vi "motor_control.vi"(6 "Drive Motor Setpoint":fxp<+/-,16,32>, 7 "Steer Motor Setpoint":fxp<+/-,16,32>) -> (0 "Wheel Position 2":i32, 1 "Desired Drive Motor Speed":fxp<+/-,16,32>, 2 "Wheel Position":i32, 3 "Desired Steer Motor Speed":fxp<+/-,16,32>)   [LabVIEW 2009]
uses:
  <vilib>/Platform/TimedLoop/XDataNode/XDataNode.xnode
  <vilib>/Platform/TimedLoop/XDataNode/loadlvalarms.vi
  <vilib>/Platform/TimedLoop/XDataNode/timing_clust.ctl
  <vilib>/Platform/TimedLoop/XDataNode/nitl_modes.ctl
  <vilib>/Platform/TimedLoop/XDataNode/wakeup.ctl
  <vilib>/eio/EIONode/EIONode.xnode
  <vilib>/rvi/eio/nirviEIOImplementation/nirviEIOImplementation.xnode
  <vilib>/rvi/eio/common/nirviEmuTemplateMethod_noerrors.vi
  <vilib>/rvi/eio/common/nirviEmuClasses.ctl
  <vilib>/addons/control/pid/fpga.llb/XNode/niFpgaPID.xnode
  <vilib>/Platform/TimedLoop/XDataNode/XDNodeRunTimeDep.lvlib
panel:
  in  "M1 Reset Position 2":bool
  in  "M1 Reset Position Value 2":i32
  out "M1 Encoder Position 2":i32
  out "M1 ticks/count 2":u32
  out "M1 Index (Z) Position 2":i32
  out "M1 counts (no reset) 2":i32
  in  "M1 Reset Position":bool
  in  "M1 Reset Position Value":i32
  out "M1 Encoder Position":i32
  out "M1 ticks/count":u32
  out "M1 Index (Z) Position":i32
  out "M1 counts (no reset)":i32
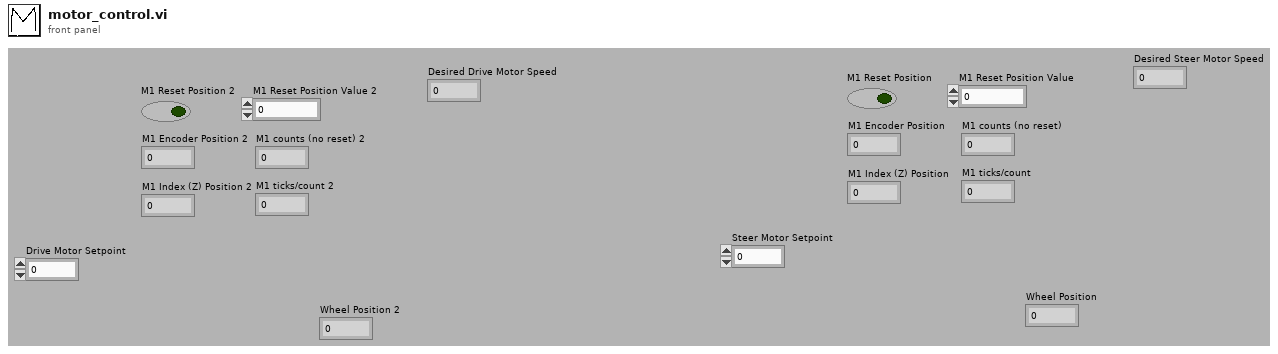
[diagram p1: front panel]
types:
  T1 = typedef "XDNodeRunTimeDep.lvlib/timing_clust.ctl" = cluster{"Expected End [f-1]":u64, "Actual End [f-1]":u64, "Finished Late? [f-1]":bool, "Expected End [i-1]":u64, "Actual End [i-1]":u64, "Finished Late? [i-1]":bool, "Expected Start [i]":u64, "Actual Start [i]":u64, "Expected Start [f]":u64, "Actual Start [f]":u64, "Source Name":string, "Structure Name":string, "Period":i64, "Deadline":i64, "Offset":i64, "Start":i64, "Priority":i32, "Timeout":i32, "Mode":T2, "Wakeup Reason":T3, "Error":errorcluster, "Source Type":string, "Secondary Source Type":string, "Global End Time":u64, "Global Start Time":u64, "Frame Duration":u64, "Iteration Duration":u64, "Assigned CPU":i32, "I/O Scan Engine Mode":u32}
  T2 = typedef "XDNodeRunTimeDep.lvlib/nitl_modes.ctl" = enum32{"No Change", "Process missed periods, maintain original phase", "Discard missed periods, maintain original phase", "Process missed periods, ignore original phase", "Discard missed periods, ignore original phase"}
  T3 = typedef "XDNodeRunTimeDep.lvlib/wakeup.ctl" = enum32{"Normal", "Aborted", "Asynchronous wakeup", "Timing source error", "Timed loop error", "Timeout"}
  T4 = cluster{"proportional gain (Kc)":i16, "integral gain (Kc*Ts/Ti)":i16, "derivative gain (Kc*Td/Ts)":i16}
  T5 = typedef "nirviEmuClasses.ctl" = enum16{"IO Read", "IO Write", "Method", "Property Read", "Property Write"}
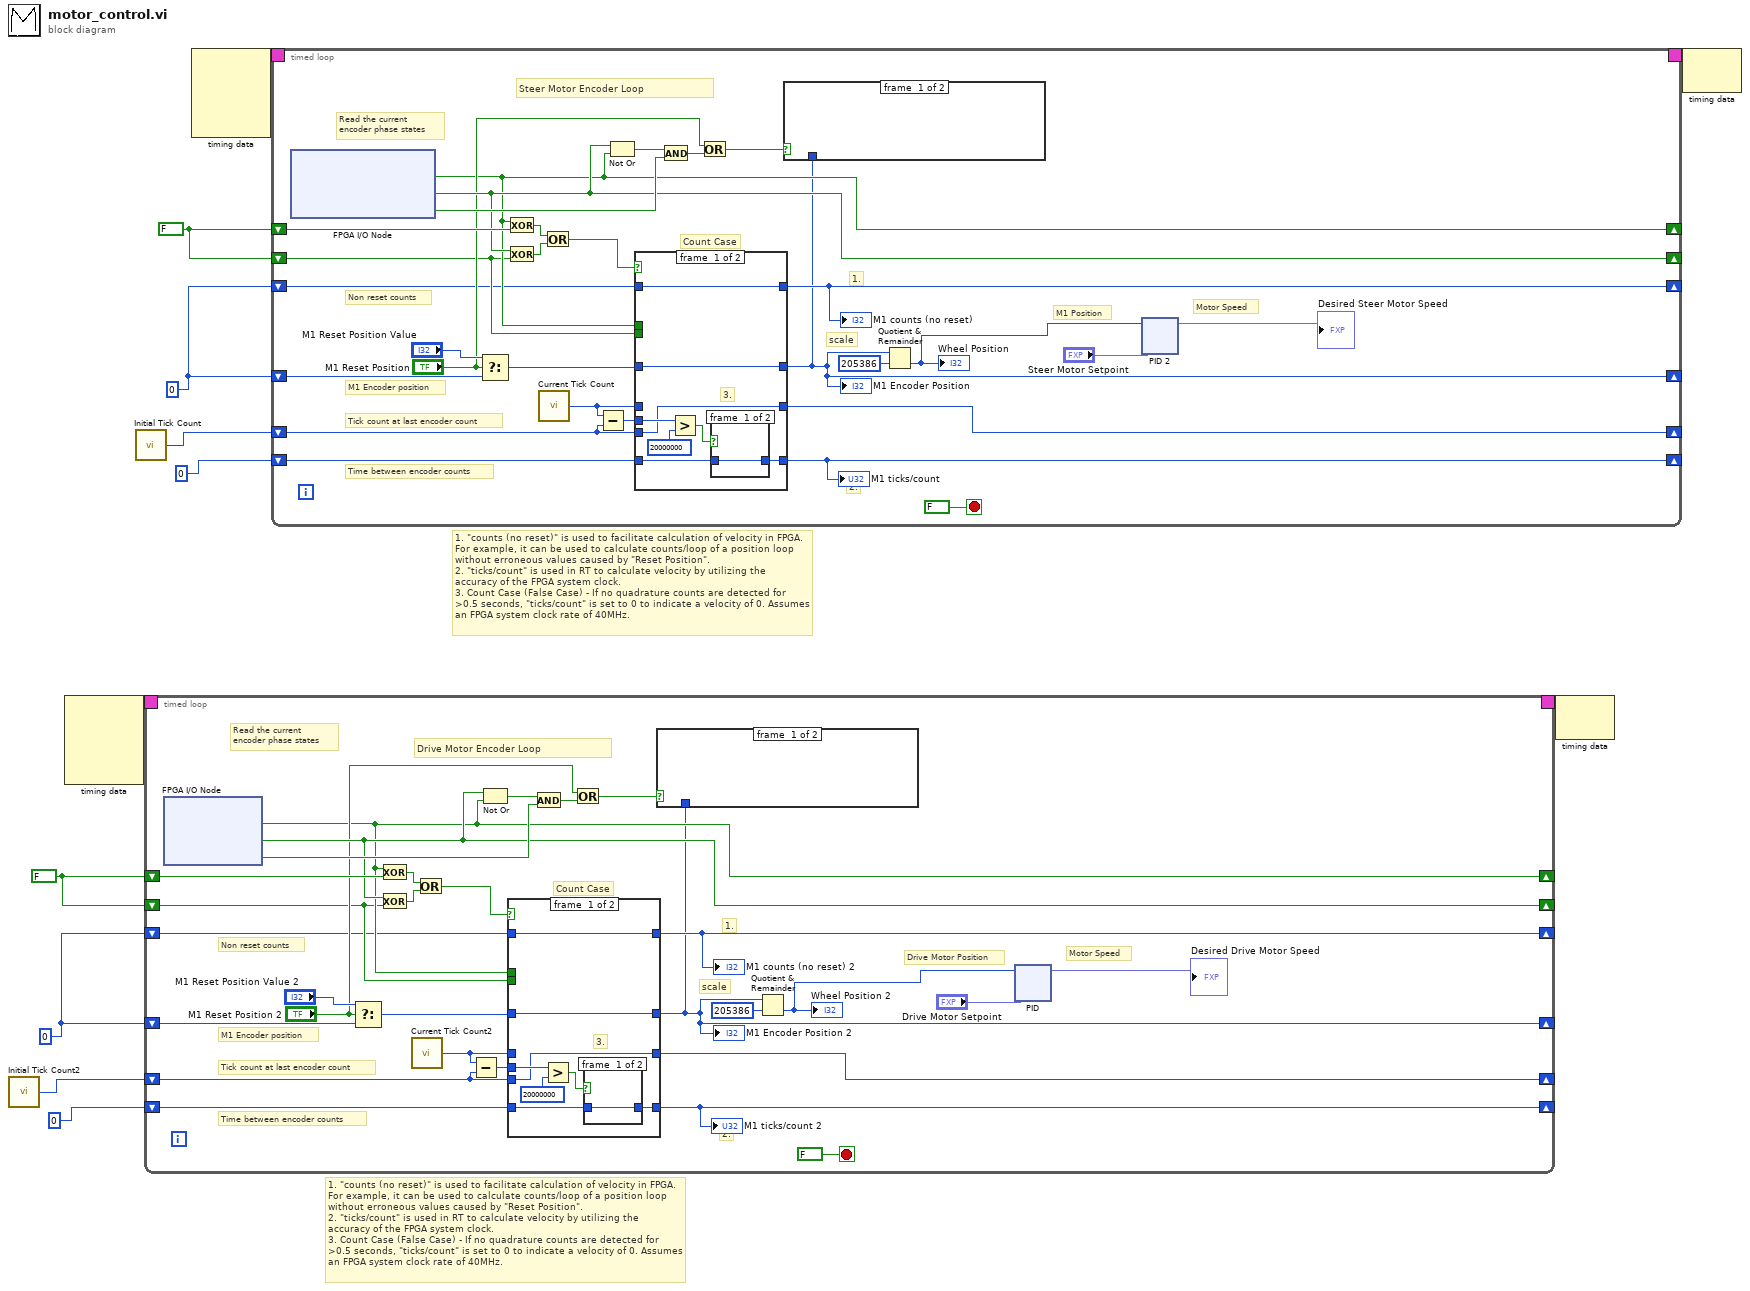
[diagram p0: block diagram]
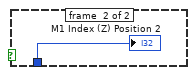
[diagram p2: hidden frame]
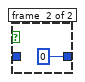
[diagram p3: hidden frame]
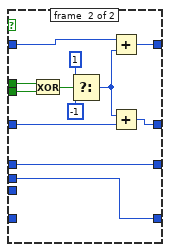
[diagram p4: hidden frame]
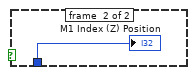
[diagram p5: hidden frame]
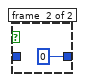
[diagram p6: hidden frame]
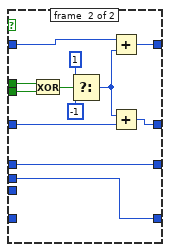
[diagram p7: hidden frame]
diagram:
  w1 = 0 ("Reset Position Value")
  w4 = FALSE ("Encoder Phase A")
  w7 = 0 ("Reset Position Value")
  w10 = FALSE ("Encoder Phase A")
  # "1. \"counts (no reset)\" is used to facilitate calculation of velocity in FPGA.\nFor example, it can be used to calculate counts/loop of a position loop\nwithout erroneous values caused by \"Reset Position\". \n2. \"ticks/count\" is used in RT to calculate velocity by utilizing the\naccuracy of the FPGA system clock.\n3. Count Case (False Case) - If no quadrature counts are detected for\n>0.5 seconds, \"ticks/count\" is set to 0 to indicate a velocity of 0. Assumes\nan FPGA system clock rate of 40MHz."
  # "1. \"counts (no reset)\" is used to facilitate calculation of velocity in FPGA.\nFor example, it can be used to calculate counts/loop of a position loop\nwithout erroneous values caused by \"Reset Position\". \n2. \"ticks/count\" is used in RT to calculate velocity by utilizing the\naccuracy of the FPGA system clock.\n3. Count Case (False Case) - If no quadrature counts are detected for\n>0.5 seconds, \"ticks/count\" is set to 0 to indicate a velocity of 0. Assumes\nan FPGA system clock rate of 40MHz."
  n1 = call "Initial Tick Count2"() -> ("Tick Count(Ticks)"=w3:u32)
  n2 = node-c288() -> (w6:T1)  [unwired: 4 in]
  n3 = call "Initial Tick Count"() -> ("Tick Count(Ticks)"=w9:u32)
  n4 = timed-loop {
    shift-right: [w24] -> _
    shift-left: w4 -> [w41]
    shift-right: [w29] -> _
    shift-left: w4 -> [w23]
    shift-right: [w16] -> _
    shift-left: w1 -> [w38]
    shift-right: [w34] -> _
    shift-left: w3 -> [w19]
    shift-right: [w33] -> _
    shift-left: u32 0 -> [w32]
    timing: w6 -> [_]
    timing-out: [_] -> w5
    shift-right: [w21] -> _
    shift-left: w1 -> [w22]
    stop <- FALSE stop-if-true
    # "Motor Speed"
    # "Drive Motor Position"
    # "scale"
    # "Count Case"
    # "Drive Motor Encoder Loop"
    # "2."
    # "1."
    # "Read the current\nencoder phase states"
    # "Non reset counts"
    # "M1 Encoder position"
    # "Time between encoder counts"
    # "Tick count at last encoder count"
    n5 = xnode "FPGA I/O Node"() -> ("Port8/DIO4"=w24:bool, "Port8/DIO5"=w29:bool, "Port8/DIO6"=w30:bool)  [unwired: 3 in, 3 out]
    n6 = Select(t="M1 Reset Position Value 2", s="M1 Reset Position 2", f=w38) -> (s? t:f=w36:i32)
    n7 = Exclusive Or(1:w41, 2:w24) -> (0:w40:bool)
    n8 = Exclusive Or(1:w23, 2:w29) -> (0:w39:bool)
    n9 = call "Current Tick Count2"() -> ("Tick Count(Ticks)"=w20:u32)
    n10 = Or(x=w40, y=w39) -> (x .or. y?=w37:bool)
    n11 = Subtract(x=w20, y=w19) -> (x-y=w18:u32)
    n12 = Not Or(1:w24, 2:w29) -> (0:w27:bool)
    n13 = case shown="True" w37 {
      tunnel: [w86 w94] -> w16
      tunnel: w36 -> [w86 w100]
      tunnel: w20 -> [_ w90]
      tunnel: [w81 w90] -> w34
      tunnel: w19 -> [w81 _]
      tunnel: [w79 w89] -> w33
      tunnel: w32 -> [w80 _]
      tunnel: w24 -> [_ w96]
      tunnel: w23 -> [_ w95]
      tunnel: [w85 w92] -> w21
      tunnel: w22 -> [w85 w91]
      tunnel: w18 -> [w82 w89]
      frame #0 {
        # "3."
        n14 = Greater?(x=w82, y=u32 20000000 ("x")) -> (0:w83:bool)
        n15 = case shown="False" w83 {
          tunnel: [w87 u32 0] -> w79
          tunnel: w80 -> [w87 _]
          frame #0 {
          }
          frame #1 {
          }
        }
      }
      frame #1 {
        n16 = Exclusive Or(1:w95, 2:w96) -> (0:w97:bool)
        n17 = Select(t=1 ("16 bit"), s=w97, f=-1 ("16 bit")) -> (s? t:f=w93:i32)
        n18 = Add(x=w91, y=w93) -> (x+y=w92:i32)
        n19 = Add(x=w93, y=w100) -> (x+y=w94:i32)
      }
    }
    "M1 Encoder Position 2" <- w16
    "M1 ticks/count 2" <- w33
    "M1 counts (no reset) 2" <- w21
    n20 = And(x=w27, y=w30) -> (x .and. y?=w28:bool)
    n21 = Or(x="M1 Reset Position 2", y=w28) -> (x .or. y?=w26:bool)
    n22 = case shown="True" w26 {
      tunnel: w16 -> [_ w78]
      frame #0 {
      }
      frame #1 {
        "M1 Index (Z) Position 2" <- w78
      }
    }
    n23 = Quotient & Remainder(x=w16, y=205386) -> (floor(x/y)=w15:i32)  [unwired: 1 out]
    "Wheel Position 2" <- w15
    n24 = xnode ("PID")("process variable"=w15, "setpoint"="Drive Motor Setpoint") -> ("output"=→"Desired Drive Motor Speed":fxp<+/-,16,32>)  [unwired: 3 in]
  }
  n25 = node-c288() -> (w12:T1)  [unwired: 4 in]
  n26 = timed-loop {
    shift-right: [w171] -> _
    shift-left: w10 -> [w188]
    shift-right: [w176] -> _
    shift-left: w10 -> [w170]
    shift-right: [w163] -> _
    shift-left: w7 -> [w185]
    shift-right: [w181] -> _
    shift-left: w9 -> [w166]
    shift-right: [w180] -> _
    shift-left: u32 0 -> [w179]
    timing: w12 -> [_]
    timing-out: [_] -> w11
    shift-right: [w168] -> _
    shift-left: w7 -> [w169]
    stop <- FALSE stop-if-true
    # "Motor Speed"
    # "M1 Position"
    # "scale"
    # "Count Case"
    # "Steer Motor Encoder Loop"
    # "2."
    # "1."
    # "Read the current\nencoder phase states"
    # "Non reset counts"
    # "M1 Encoder position"
    # "Time between encoder counts"
    # "Tick count at last encoder count"
    n27 = xnode "FPGA I/O Node"() -> ("M1_encoder_PhaseA"=w171:bool, "M1_encoder_PhaseB"=w176:bool, "M1_encoder_index"=w177:bool)  [unwired: 3 in, 3 out]
    n28 = Select(t="M1 Reset Position Value", s="M1 Reset Position", f=w185) -> (s? t:f=w183:i32)
    n29 = Exclusive Or(1:w188, 2:w171) -> (0:w187:bool)
    n30 = Exclusive Or(1:w170, 2:w176) -> (0:w186:bool)
    n31 = call "Current Tick Count"() -> ("Tick Count(Ticks)"=w167:u32)
    n32 = Or(x=w187, y=w186) -> (x .or. y?=w184:bool)
    n33 = Subtract(x=w167, y=w166) -> (x-y=w165:u32)
    n34 = Not Or(1:w171, 2:w176) -> (0:w174:bool)
    n35 = case shown="True" w184 {
      tunnel: [w233 w241] -> w163
      tunnel: w183 -> [w233 w247]
      tunnel: w167 -> [_ w237]
      tunnel: [w228 w237] -> w181
      tunnel: w166 -> [w228 _]
      tunnel: [w226 w236] -> w180
      tunnel: w179 -> [w227 _]
      tunnel: w171 -> [_ w243]
      tunnel: w170 -> [_ w242]
      tunnel: [w232 w239] -> w168
      tunnel: w169 -> [w232 w238]
      tunnel: w165 -> [w229 w236]
      frame #0 {
        # "3."
        n36 = Greater?(x=w229, y=u32 20000000 ("x")) -> (0:w230:bool)
        n37 = case shown="False" w230 {
          tunnel: [w234 u32 0] -> w226
          tunnel: w227 -> [w234 _]
          frame #0 {
          }
          frame #1 {
          }
        }
      }
      frame #1 {
        n38 = Exclusive Or(1:w242, 2:w243) -> (0:w244:bool)
        n39 = Select(t=1 ("16 bit"), s=w244, f=-1 ("16 bit")) -> (s? t:f=w240:i32)
        n40 = Add(x=w238, y=w240) -> (x+y=w239:i32)
        n41 = Add(x=w240, y=w247) -> (x+y=w241:i32)
      }
    }
    "M1 Encoder Position" <- w163
    "M1 ticks/count" <- w180
    "M1 counts (no reset)" <- w168
    n42 = And(x=w174, y=w177) -> (x .and. y?=w175:bool)
    n43 = Or(x="M1 Reset Position", y=w175) -> (x .or. y?=w173:bool)
    n44 = case shown="True" w173 {
      tunnel: w163 -> [_ w225]
      frame #0 {
      }
      frame #1 {
        "M1 Index (Z) Position" <- w225
      }
    }
    n45 = Quotient & Remainder(x=w163, y=205386) -> (floor(x/y)=w162:i32)  [unwired: 1 out]
    "Wheel Position" <- w162
    n46 = xnode ("PID 2")("process variable"=w162, "setpoint"="Steer Motor Setpoint") -> ("output"=→"Desired Steer Motor Speed":fxp<+/-,16,32>)  [unwired: 3 in]
  }
  n47 = node-c288(w5) -> ()  [unwired: 1 out]
  n48 = node-c288(w11) -> ()  [unwired: 1 out]
